vi "NL-Modell-Doppelpendel.vi"(0 "Kraft (N)":dbl, 1 "Position_t0":dbl, 2 "Winkel1_t0":dbl, 3 "Winkelg.1_t0":dbl, 4 "Winkel2_t0":dbl, 5 "Winkelg.2_t0":dbl) -> (14 "Position":dbl, 15 "Winkel1":dbl, 16 "Winkel 2":dbl, 17 "Geschwindigkeit":dbl, 18 "Winkelg.1":dbl, 19 "Winkelg.2":dbl)   [LabVIEW 2014]
uses:
  <vilib>/Simulation/Implementation/Shared/SIMSCR Execution Mode.ctl
  <vilib>/Simulation/Scripting/Companion Diagram/SimConfigNode/SimParams.ctl
  <vilib>/Simulation/Scripting/Companion Diagram/SimConfigNode/_simSolvers.ctl
  <vilib>/Simulation/Param Hierarchy/Typedefs/SIMPH Param Control Actions.ctl
  <vilib>/Simulation/Implementation/Shared/SIM limit type.ctl
  <vilib>/Simulation/Implementation/Shared/NILVSim_ParamChanged.vi
  <vilib>/Simulation/Implementation/Shared/NILVSIM_BeginStep.vi
  <vilib>/Simulation/ContinuousLinear/Implementation/NILVSim Integrator new.llb/SIM Integrator distributor (scalar).vi
  <vilib>/Simulation/ContinuousLinear/Implementation/NILVSim Integrator new.llb/SIM Integrator collector (scalar).vi
  <vilib>/Simulation/Implementation/Shared/NILVSim_Manager.vi
  <vilib>/Utility/error.llb/Clear Errors.vi
  <vilib>/Simulation/Implementation/Shared/NILVSim_FinalizeModel.vi
  <vilib>/Simulation/Implementation/Shared/SIM Unbundle Sim Info.vi
  <vilib>/Simulation/Implementation/Shared/SIMSH Read Queue.vi
  <vilib>/Simulation/Implementation/Shared/NILVSim_Initialize.vi
  <vilib>/Simulation/Utility/Implementation/NILVSim Get Time and IsAcceptedStep.vi
  <vilib>/Simulation/Implementation/Shared/NILVSim_GetModelError.vi
  <vilib>/Simulation/Implementation/Shared/SIM SimErrorHandler.vi
  <vilib>/Simulation/Implementation/Shared/SIM Bundle Sim Info.vi
  <vilib>/Simulation/Scripting/Companion Diagram/SimConfigNode/SimDog.xnode
  <vilib>/Simulation/ContinuousLinear/Implementation/NILVSim Integrator new.llb/SIM Integrator (scalar).vi
  <vilib>/Simulation/Implementation/XNodeFramework/SimXNode/SimX.xnode
  <vilib>/Simulation/Implementation/Shared/NI_SIM_Implementation.lvlib
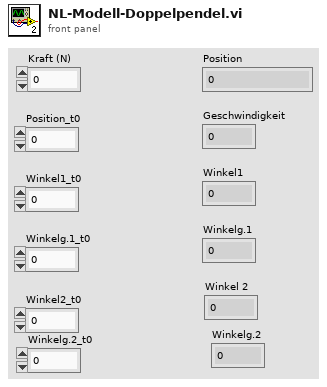
[diagram p1: front panel]
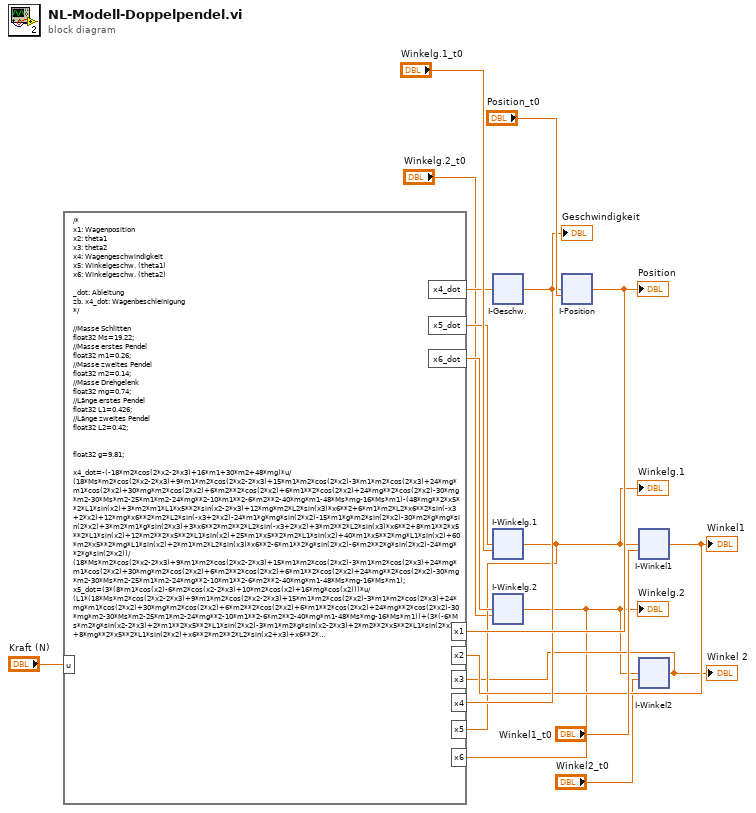
[diagram p0: block diagram]
diagram:
  n1 = formula code="/*\nx1: Wagenposition\nx2: theta1\nx3: theta2\nx4: Wagengeschwindigkeit \nx5: Winkelgeschw. (theta1)\nx6: Winkelgeschw. (theta2)\n\n_dot: Ableitung\nzb. x4_dot: Wagenbeschleinigung\n*/\n\n//Masse Schlitten\nfloat32 Ms=19.22;\n//Masse erstes Pendel\nfloat32 m1=0.26;\n//Masse zweites Pendel\nfloat32 m2=0.14;\n//Masse Drehgelenk\nfloat32 mg=0.74;\n//Länge erstes Pendel\nfloat32 L1=0.426;\n//Länge zweites Pendel\nfloat32 L2=0.42;\n\n\nfloat32 g=9.81;\n\nx4_dot=-(-18*m2*cos(2*x2-2*x3)+16*m1+30*m2+48*mg)*u/(18*Ms*m2*cos(2*x2-2*x3)+9*m1*m2*cos(2*x2-2*x3)+15*m1*m2*cos(2*x2)-3*m1*m2*cos(2*x3)+24*mg*m1*cos(2*x2)+30*mg*m2*cos(2*x2)+6*m2**2*cos(2*x2)+6*m1**2*cos(2*x2)+24*mg**2*cos(2*x2)-30*mg*m2-30*Ms*m2-25*m1*m2-24*mg**2-10*m1**2-6*m2**2-40*mg*m1-48*Ms*mg-16*Ms*m1)-(48*mg**2*x5**2*L1*sin(x2)+3*m2*m1*L1*x5**2*sin(x2-2*x3)+12*mg*m2*L2*sin(x3)*x6**2+6*m1*m2*L2*x6**2*sin(-x3+2*x2)+12*mg*x6**2*m2*L2*sin(-x3+2*x2)-24*m1*g*mg*sin(2*x2)-15*m1*g*m2*sin(2*x2)-30*m2*g*mg*sin(2*x2)+3*m2*m1*g*sin(2*x3)+3*x6**2*m2**2*L2*sin(-x3+2*x2)+3*m2**2*L2*sin(x3)*x6**2+8*m1**2*x5**2*L1*sin(x2)+12*m2**2*x5**2*L1*sin(x2)+25*m1*x5**2*m2*L1*sin(x2)+40*m1*x5**2*mg*L1*sin(x2)+60*m2*x5**2*mg*L1*sin(x2)+2*m1*m2*L2*sin(x3)*x6**2-6*m1**2*g*sin(2*x2)-6*m2**2*g*sin(2*x2)-24*mg**2*g*sin(2*x2))/(18*Ms*m2*cos(2*x2-2*x3)+9*m1*m2*cos(2*x2-2*x3)+15*m1*m2*cos(2*x2)-3*m1*m2*cos(2*x3)+24*mg*m1*cos(2*x2)+30*mg*m2*cos(2*x2)+6*m2**2*cos(2*x2)+6*m1**2*cos(2*x2)+24*mg**2*cos(2*x2)-30*mg*m2-30*Ms*m2-25*m1*m2-24*mg**2-10*m1**2-6*m2**2-40*mg*m1-48*Ms*mg-16*Ms*m1);\nx5_dot=(3*(8*m1*cos(x2)-6*m2*cos(x2-2*x3)+10*m2*cos(x2)+16*mg*cos(x2)))*u/(L1*(18*Ms*m2*cos(2*x2-2*x3)+9*m1*m2*cos(2*x2-2*x3)+15*m1*m2*cos(2*x2)-3*m1*m2*cos(2*x3)+24*mg*m1*cos(2*x2)+30*mg*m2*cos(2*x2)+6*m2**2*cos(2*x2)+6*m1**2*cos(2*x2)+24*mg**2*cos(2*x2)-30*mg*m2-30*Ms*m2-25*m1*m2-24*mg**2-10*m1**2-6*m2**2-40*mg*m1-48*Ms*mg-16*Ms*m1))+(3*(-6*Ms*m2*g*sin(x2-2*x3)+2*m1**2*x5**2*L1*sin(2*x2)-3*m1*m2*g*sin(x2-2*x3)+2*m2**2*x5**2*L1*sin(2*x2)+8*mg**2*x5**2*L1*sin(2*x2)+x6**2*m2**2*L2*sin(x2+x3)+x6**2*m2**2*L2*sin(x2-x3)-20*mg*g*m2*sin(x2)-24*mg*g*m1*sin(x2)-16*Ms*g*mg*sin(x2)-10*Ms*g*m2*sin(x2)-8*Ms*g*m1*sin(x2)-15*m1*g*m2*sin(x2)-4*g*m2**2*sin(x2)-16*g*mg**2*sin(x2)-8*g*m1**2*sin(x2)+5*m1*x5**2*m2*L1*sin(2*x2)+3*m2*m1*L1*x5**2*sin(2*x2-2*x3)+10*m2*x5**2*mg*L1*sin(2*x2)+6*Ms*m2*L1*x5**2*sin(2*x2-2*x3)+8*m1*x5**2*mg*L1*sin(2*x2)+4*mg*x6**2*m2*L2*sin(x2+x3)+4*mg*x6**2*m2*L2*sin(x2-x3)+8*Ms*m2*L2*x6**2*sin(x2-x3)+2*m1*m2*L2*x6**2*sin(x2+x3)+6*m1*m2*L2*x6**2*sin(x2-x3)))/(L1*(18*Ms*m2*cos(2*x2-2*x3)+9*m1*m2*cos(2*x2-2*x3)+15*m1*m2*cos(2*x2)-3*m1*m2*cos(2*x3)+24*mg*m1*cos(2*x2)+30*mg*m2*cos(2*x2)+6*m2**2*cos(2*x2)+6*m1**2*cos(2*x2)+24*mg**2*cos(2*x2)-30*mg*m2-30*Ms*m2-25*m1*m2-24*mg**2-10*m1**2-6*m2**2-40*mg*m1-48*Ms*mg-16*Ms*m1));\nx6_dot=-(3*(12*mg*cos(-x3+2*x2)+6*m1*cos(-x3+2*x2)-2*m1*cos(x3)+12*m2*cos(-x3+2*x2)-12*cos(x3)*mg-12*m2*cos(x3)))*u/(L2*(18*Ms*m2*cos(2*x2-2*x3)+9*m1*m2*cos(2*x2-2*x3)+15*m1*m2*cos(2*x2)-3*m1*m2*cos(2*x3)+24*mg*m1*cos(2*x2)+30*mg*m2*cos(2*x2)+6*m2**2*cos(2*x2)+6*m1**2*cos(2*x2)+24*mg**2*cos(2*x2)-30*mg*m2-30*Ms*m2-25*m1*m2-24*mg**2-10*m1**2-6*m2**2-40*mg*m1-48*Ms*mg-16*Ms*m1))-(3*(m1**2*L1*x5**2*sin(x2+x3)+3*m1**2*L1*x5**2*sin(x2-x3)-6*m1*m2*g*sin(-x3+2*x2)-6*mg*m1*g*sin(-x3+2*x2)-12*Ms*mg*g*sin(-x3+2*x2)-12*Ms*m2*g*sin(-x3+2*x2)-6*Ms*m1*g*sin(-x3+2*x2)+2*mg*m1*g*sin(x3)+12*Ms*m2*g*sin(x3)+12*Ms*mg*g*sin(x3)+2*Ms*m1*g*sin(x3)+2*m1*m2*g*sin(x3)-3*m1**2*g*sin(-x3+2*x2)-m1**2*g*sin(x3)+3*m1*m2*L2*x6**2*sin(2*x2-2*x3)+m1*m2*L2*x6**2*sin(2*x3)+6*Ms*m2*L2*x6**2*sin(2*x2-2*x3)+10*m2*m1*L1*x5**2*sin(x2-x3)+2*mg*m1*L1*x5**2*sin(x2+x3)+10*mg*m1*L1*x5**2*sin(x2-x3)+2*m2*m1*L1*x5**2*sin(x2+x3)+8*Ms*m1*L1*x5**2*sin(x2-x3)+24*Ms*mg*L1*x5**2*sin(x2-x3)+24*Ms*m2*L1*x5**2*sin(x2-x3)))/(L2*(18*Ms*m2*cos(2*x2-2*x3)+9*m1*m2*cos(2*x2-2*x3)+15*m1*m2*cos(2*x2)-3*m1*m2*cos(2*x3)+24*mg*m1*cos(2*x2)+30*mg*m2*cos(2*x2)+6*m2**2*cos(2*x2)+6*m1**2*cos(2*x2)+24*mg**2*cos(2*x2)-30*mg*m2-30*Ms*m2-25*m1*m2-24*mg**2-10*m1**2-6*m2**2-40*mg*m1-48*Ms*mg-16*Ms*m1));" ("Formelknoten 2")("x1"=w8, "x2"=w6, "x4"=w7, "x3"=w2, "x5"=w5, "x6"=w1, "u"="Kraft (N)") -> ("x4_dot"=w11:dbl, "x5_dot"=w10:dbl, "x6_dot"=w9:dbl)
  n2 = xnode "I-Geschw."("input"=w11) -> ("output"=w7:dbl)  [unwired: 9 in, 2 out]
  "Geschwindigkeit" <- w7
  n3 = xnode "I-Winkelg.1"("input"=w10, "initial condition"="Winkelg.1_t0") -> ("output"=w5:dbl)  [unwired: 8 in, 2 out]
  "Winkelg.1" <- w5
  n4 = xnode "I-Winkelg.2"("input"=w9, "initial condition"="Winkelg.2_t0") -> ("output"=w1:dbl)  [unwired: 8 in, 2 out]
  "Winkelg.2" <- w1
  n5 = xnode "I-Position"("input"=w7, "initial condition"="Position_t0") -> ("output"=w8:dbl)  [unwired: 8 in, 2 out]
  "Position" <- w8
  n6 = xnode "I-Winkel1"("input"=w5, "initial condition"="Winkel1_t0") -> ("output"=w6:dbl)  [unwired: 8 in, 2 out]
  "Winkel1" <- w6
  n7 = xnode "I-Winkel2"("input"=w1, "initial condition"="Winkel2_t0") -> ("output"=w2:dbl)  [unwired: 8 in, 2 out]
  "Winkel 2" <- w2
